vi "ListAvailablePackagesInFeed.vi"(8 "Error In":errorcluster, 10 "Log File Path (*.csv)":path, 11 "FeedURL(s)":string[](array[string])) -> (0 "Error Out":errorcluster, 3 "PackageMeta":T1[](array[typedef]))   [LabVIEW 2019, in "CEPM.lvlib"]
uses:
  CEPM.lvlib
  Typedefs/PackageMeta.ctl
  <vilib>/SLL Toolkit/SLL File IO/Spreadsheet/CSV Logger/_Typedefs/String Key Value Pair Cluster.ctl
  <vilib>/SLL Toolkit/SLL File IO/Spreadsheet/CSV Logger/SLL CSV Logger.lvclass
  <vilib>/National Instruments/NIPM API (Beta)/NIPM_API.lvlib
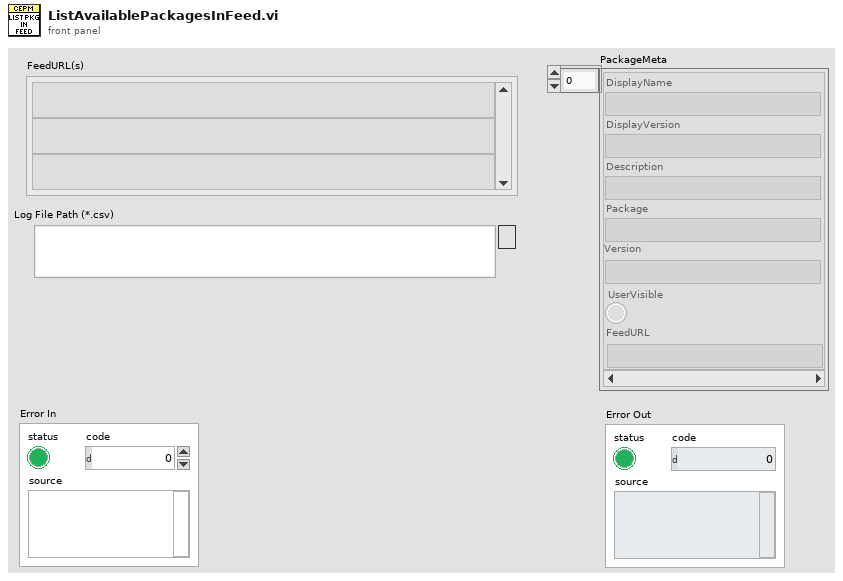
[diagram p1: front panel]
types:
  T1 = typedef "CEPM.lvlib/PackageMeta.ctl" = cluster{"DisplayName":string, "DisplayVersion":string, "Description":string, "Package":string, "Version":string, "UserVisible":bool, "FeedURL":string}
  T2 = typedef "SLL Spreadsheet.lvlib/SLL CSV Logger.lvclass/String Key Value Pair Cluster.ctl" = cluster{"Key":string, "Value":string}
  T3 = typedef "NIPM_API.lvlib/feed.ctl" = cluster{"Name":string, "URI":string}
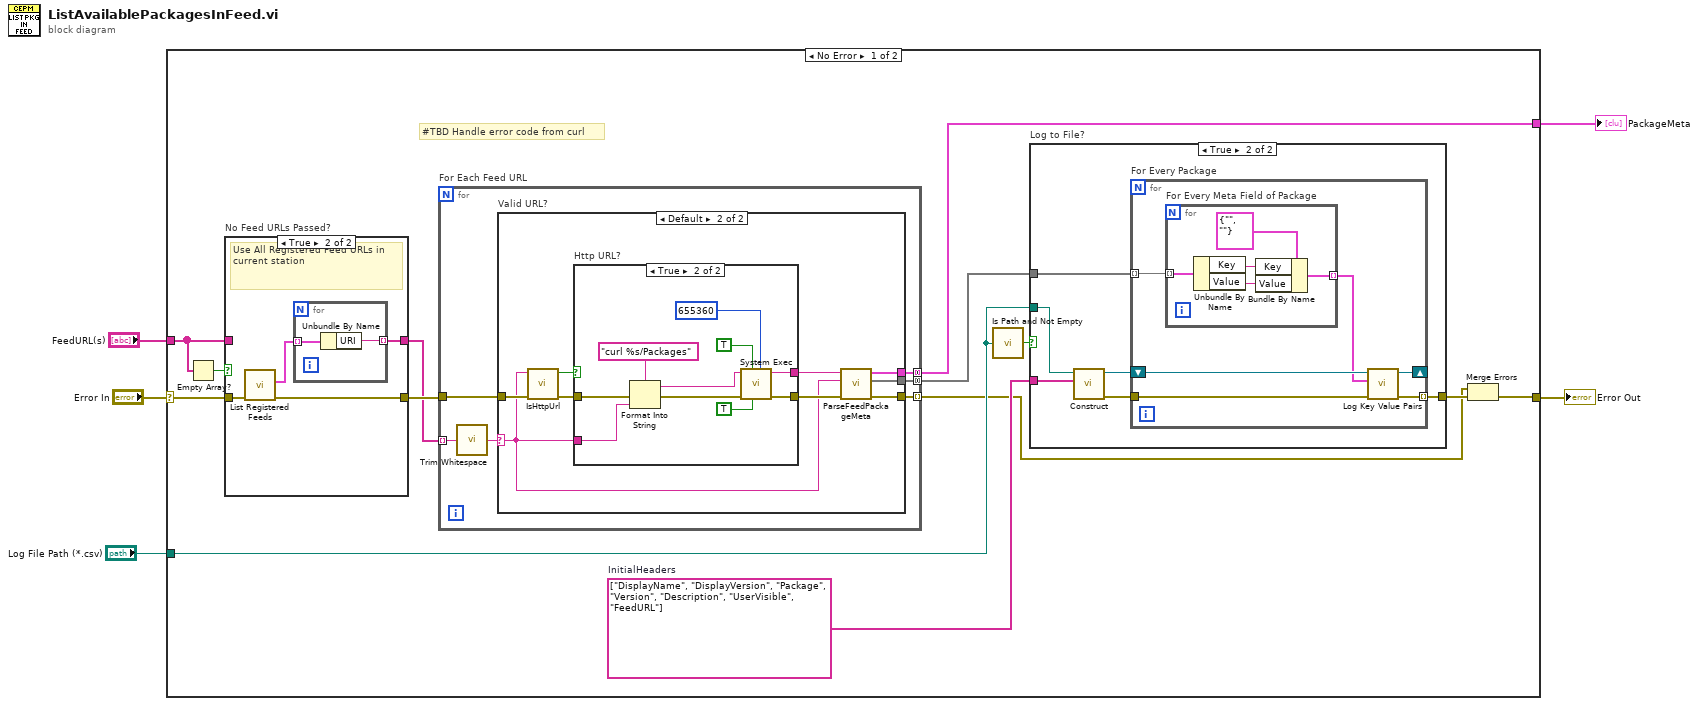
[diagram p0: block diagram]
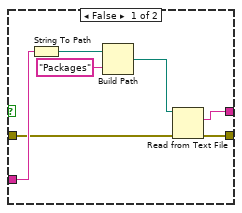
[diagram p5: hidden frame]
diagram:
  n1 = case shown="No Error" "Error In" {
    selector: "Error In" -> [w18 w77]
    tunnel: [w11 w77] -> w4
    tunnel: "FeedURL(s)" -> [w7 _]
    tunnel: [w17 _] -> w2
    tunnel: "Log File Path (*.csv)" -> [w14 _]
    frame No Error {
      w12 = string[] ["DisplayName", "DisplayVersion", "Package", "Version", "Description", "UserVisible", "FeedURL"]  # InitialHeaders
      # "#TBD Handle error code from curl"
      n2 = Empty Array?(array=w7) -> (empty?=w8:bool)
      n3 = case "No Feed URLs Passed?" shown="True" w8 {
        tunnel: w18 -> [w19 w24]
        tunnel: [w19 w23] -> w9
        tunnel: w7 -> [w20 _]
        tunnel: [w20 w21] -> w6
        frame False {
        }
        frame True {
          # "Use All Registered Feed URLs in current station"
          n4 = call <vilib>:"List Registered Feeds.vi"("error in"=w24) -> ("error out"=w23:errorcluster, "registered feeds"=w22:T3[])  [unwired: 9 in]
          n5 = for {
            tunnel: w22 -> [w26] mode=indexing
            tunnel: [w25] -> w21 mode=indexing
            n6 = Unbundle By Name(w26) -> ("URI"=w25:string)
          }
        }
      }
      n7 = for "For Each Feed URL" {
        tunnel: [w48] -> w17 mode=concatenating
        tunnel: [w47] -> w16 mode=concatenating
        tunnel: w6 -> [w45] mode=indexing
        tunnel: w9 -> [w49]
        tunnel: [w46] -> w10 mode=indexing
        n8 = call <vilib>:"Trim Whitespace.vi"("string"=w45) -> ("trimmed string"=w44:string)  [unwired: 1 in]
        n9 = case "Valid URL?" shown="Default" w44 {
          selector: w44 -> [_ w52]
          tunnel: w49 -> [w50 w54]
          tunnel: [_ w57] -> w48
          tunnel: [_ w56] -> w47
          tunnel: [w50 w55] -> w46
          frame "" {
          }
          frame Default {
            n10 = call "IsHttpUrl.vi"("Error In"=w54, "URL"=w52) -> ("Error Out"=w53:errorcluster, "Web URL?"=w51:bool)  [unwired: 8 in]
            n11 = case "Http URL?" shown="True" w51 {
              tunnel: [w63 w70] -> w59
              tunnel: [w60 w69] -> w58
              tunnel: w53 -> [w62 w68]
              tunnel: w52 -> [w66 w67]
              frame False {
                n12 = String To Path(string=w66) -> (path=w65:path)
                n13 = Build Path(base path=w65, name or relative path="Packages") -> (appended path=w61:path)
                n14 = Read from Text File(file (use dialog)=w61, error in=w62) -> (text=w60:string, error out=w63:errorcluster)  [unwired: 2 in, 2 out]
              }
              frame True {
                n15 = Format Into String(format string="curl %s/Packages", error in=w68, w67) -> (resulting string=w74:string, error out=w76:errorcluster)  [unwired: 1 in]
                n16 = call <vilib>:"System Exec.vi"("expected output size  (4096)"=u32 655360, "run minimized? (F)"=TRUE, "wait until completion? (T)"=TRUE, "error in (no error)"=w76, "command line"=w74) -> ("error out"=w70:errorcluster, "standard output"=w69:string)  [unwired: 3 in, 2 out]
              }
            }
            n17 = call "ParseFeedPackageMeta.vi"("Error In"=w59, "FeedURL"=w52, "FeedPackageMeta"=w58) -> ("Error Out"=w55:errorcluster, "PackageMetaMap"=w56:map{string, string}[], "PackageMeta"=w57:T1[])  [unwired: 6 in]
          }
        }
      }
      n18 = call <vilib>:"Is Path and Not Empty.vi"("path"=w14) -> ("Is Path and Not Empty?"=w15:bool)  [unwired: 4 in]
      n19 = case "Log to File?" shown="True" w15 {
        tunnel: w16 -> [_ w32]
        tunnel: w14 -> [_ w31]
        tunnel: [_ w28] -> w13
        tunnel: w12 -> [_ w27]
        frame False {
        }
        frame True {
          n20 = call <vilib>:"Construct.vi"("Starter Headers[]"=w27, "File Path"=w31) -> ("error out"=w30:errorcluster, "SLL CSV Logger out"=w29:refnum<class "SLL CSV Logger.lvclass">)  [unwired: 8 in]
          n21 = for "For Every Package" {
            tunnel: w32 -> [w38] mode=indexing
            shift-right: [w36] -> _
            shift-left: w29 -> [w37]
            tunnel: w30 -> [w34]
            tunnel: [w33] -> w28 mode=indexing
            n22 = for "For Every Meta Field of Package" {
              tunnel: w38 -> [w43] mode=indexing
              tunnel: [w39] -> w35 mode=indexing
              n23 = Unbundle By Name(w43) -> ("Key"=w41:string, "Value"=w40:string)
              n24 = Bundle By Name(cluster=T2 {"Key"="", "Value"=""} ("Cluster"), "Key"=w41, "Value"=w40) -> (w39:T2)
            }
            n25 = call <vilib>:"Log Key Value Pairs.vi"("error in (no error)"=w34, "String Key Value Pairs"=w35, "SLL Spreadsheet Logger in"=w37) -> ("error out"=w33:errorcluster, "SLL Spreadsheet Logger out"=w36:refnum<class "SLL CSV Logger.lvclass">)  [unwired: 7 in]
          }
        }
      }
      n26 = Merge Errors(w10, w13) -> (w11:errorcluster)
    }
    frame Error {
    }
  }
  "Error Out" <- w4
  "PackageMeta" <- w2
